vi "Pre Launch Init.vi"(11 "GUI Señal Actualizable in":refnum<class "GUI Señal Actualizable.lvclass">) -> (0 "error out":errorcluster, 3 "GUI Señal Actualizable out":refnum<class "GUI Señal Actualizable.lvclass">)   [LabVIEW 2020, in "GUI Señal Actualizable.lvlib" / "GUI Señal Actualizable.lvclass"]
doc: "(<B>Filename</B>: Actor Framework.lvlib:Actor.lvclass:Pre Launch Init.vi)\n\nDefines behavior that occurs after the Launch Nested Actor method is invoked but before the actor's Actor Core method begins running.\n\nBy default, this method does nothing. A descendant class may override it to define behavior."
uses:
  <vilib>/ActorFramework/Actor/Actor.lvclass
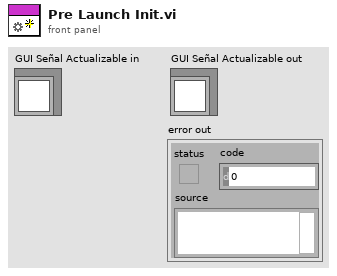
[diagram p1: front panel]
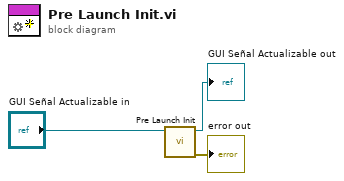
[diagram p0: block diagram]
diagram:
  n1 = call-parent "Pre Launch Init.vi"("Actor in"="GUI Señal Actualizable in") -> ("error out"=→"error out":errorcluster, "Actor out"=→"GUI Señal Actualizable out":refnum<class "GUI Señal Actualizable.lvclass">)  [unwired: 9 in]
